vi "Aktualizacja ostatniego zaznaczonego położenia na mapie.vi"(6 "Pocz. poł.":T1 {"UTM"."N [m]" format="%#_10g"}, 7 "Aktualne położenie":T2 {"Szerokośc geograficzna - GPS" format="%_9f"; "Długość geograficzna - GPS" format="%_9f"; "Położenie \nrobota  UTM"."E [m]" format="%#_10g"; "Położenie \nrobota  UTM"."N [m]" format="%#_12g"}, 8 "Właściwości mapy in":T5, 9 "Mouse down coords":T3, 10 "Parametry odwzorowania Ziemi (WGS84)":cluster{"a":dbl, "b":dbl}, 11 "Picture in":refnum<vi>) -> (2 "Właściwości mapy out":T5, 3 "Pocz. poł. 2":T1 {"UTM"."N [m]" format="%#_10g"})   [LabVIEW 2012, in "Biblioteka moduł map v3.lvlib" / "Pomocnicze.lvlib"]
uses:
  Pomocnicze.lvlib
  <vilib>/Utility/miscctls.llb/LVBoundsTypeDef.ctl
  <vilib>/Utility/miscctls.llb/LVPoint32TypeDef.ctl
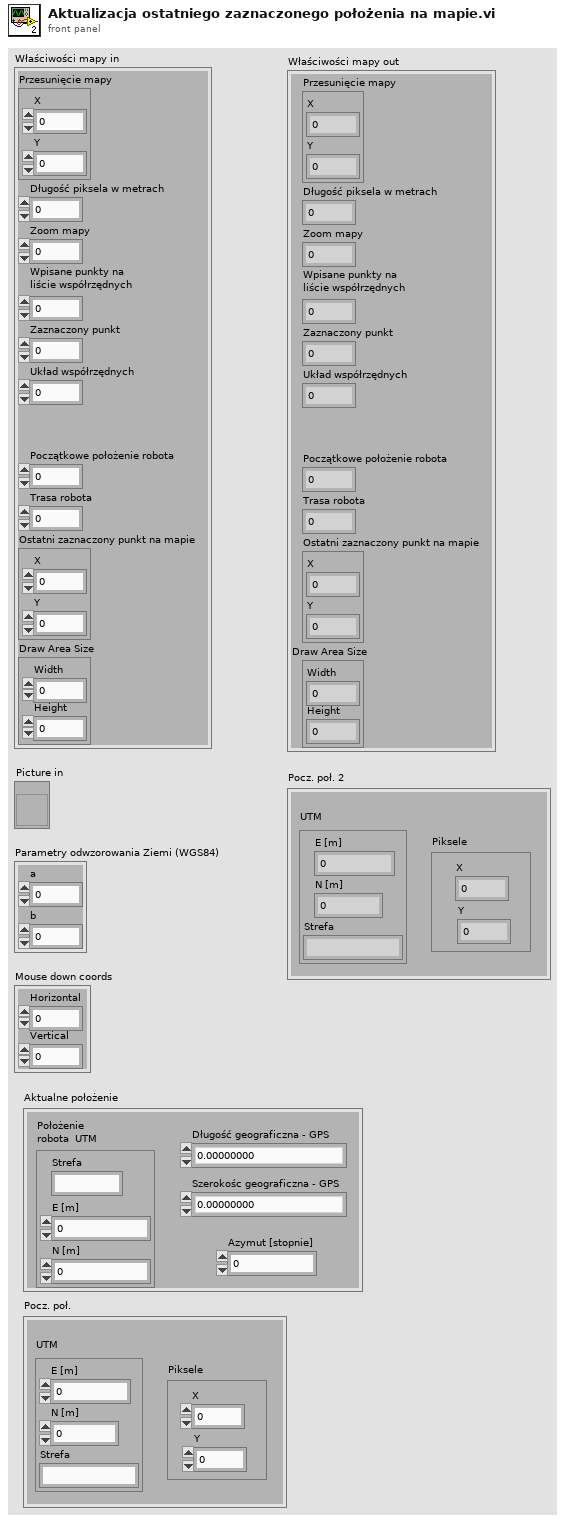
[diagram p1: front panel]
types:
  T1 = cluster{"UTM":cluster{"E [m]":ext, "N [m]":ext, "Strefa":string}, "Piksele":cluster{"X":i32, "Y":i32}}
  T2 = cluster{"Położenie \nrobota  UTM":cluster{"E [m]":ext, "N [m]":ext, "Strefa":string}, "Długość geograficzna - GPS":dbl, "Szerokośc geograficzna - GPS":dbl, "Azymut [stopnie]":dbl}
  T3 = typedef "LVPoint32TypeDef.ctl" = cluster{"Horizontal":i32, "Vertical":i32}
  T4 = typedef "LVBoundsTypeDef.ctl" = cluster{"Width":u32, "Height":u32}
  T5 = cluster{"Przesunięcie mapy":cluster{"X":i16, "Y":i16}, "Długość piksela w metrach":dbl, "Zoom mapy":sgl, "Wpisane punkty na\nliście współrzędnych":u32, "Zaznaczony punkt":u32, "Układ współrzędnych":u32, "Początkowe położenie robota":u32, "Trasa robota":u32, "Ostatni zaznaczony punkt na mapie":cluster{"X":i32, "Y":i32}, "Draw Area Size":T4}
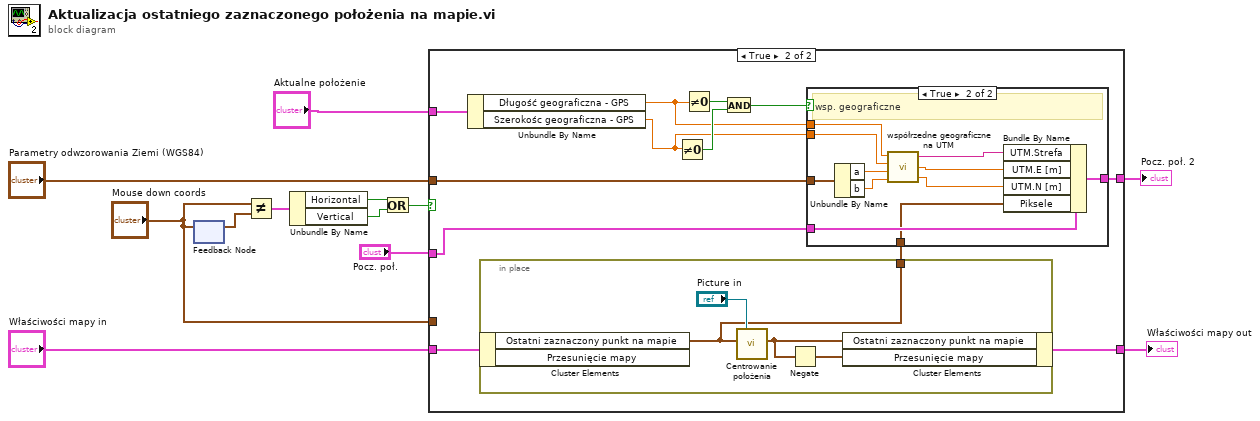
[diagram p0: block diagram]
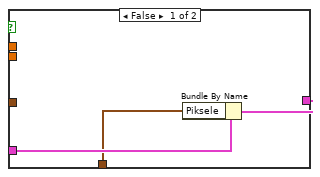
[diagram p3: hidden frame]
diagram:
  n1 = feedback #1() -> (w5:T3)  [unwired: 1 in]
  n2 = feedback-in #1("Mouse down coords") -> ()
  n3 = Not Equal?(x="Mouse down coords", y=w5) -> (x != y?=w6:cluster{"Horizontal":bool, "Vertical":bool})
  n4 = Unbundle By Name(w6) -> ("Horizontal"=w8:bool, "Vertical"=w9:bool)
  n5 = Or(x=w8, y=w9) -> (x .or. y?=w7:bool)
  n6 = case shown="True" w7 {
    tunnel: "Mouse down coords" -> [_ _]
    tunnel: "Właściwości mapy in" -> [w13 w17]
    tunnel: [w13 w19] -> w12
    tunnel: "Parametry odwzorowania Ziemi (WGS84)" -> [_ w26]
    tunnel: "Pocz. poł." -> [w14 w15]
    tunnel: [w14 w20] -> w1
    tunnel: "Aktualne położenie" -> [_ w16]
    frame False {
    }
    frame True {
      n7 = Unbundle By Name(w16) -> ("Długość geograficzna - GPS"=w21:dbl, "Szerokośc geograficzna - GPS"=w23:dbl)
      n8 = in-place {
        in-place-border: [w27] -> w18
        n9 = in-place-cluster #2(w17) -> ("Ostatni zaznaczony punkt na mapie"=w27:cluster{"X":i32, "Y":i32})  [unwired: 1 out]
        n10 = call "Centrowanie położenia.vi"("Ostatnie położenie robota"=w27, "Mapa z wprowadzonym punktem"="Picture in") -> ("Przesunięcie wycentrowane"=w28:T3)  [unwired: 9 in]
        n11 = Negate(x=w28) -> (-x=w29:T3)
        n12 = in-place-cluster #2("Ostatni zaznaczony punkt na mapie"=w28, "Przesunięcie mapy"=w29) -> (w19:T5)
      }
      n13 = Not Equal To 0?(x=w23) -> (x != 0?=w25:bool)
      n14 = Not Equal To 0?(x=w21) -> (x != 0?=w22:bool)
      n15 = And(x=w22, y=w25) -> (x .and. y?=w24:bool)
      n16 = case shown="True" w24 {
        tunnel: w26 -> [_ w44]
        tunnel: w21 -> [_ w38]
        tunnel: w23 -> [_ w37]
        tunnel: w15 -> [w33 w35]
        tunnel: [w31 w36] -> w20
        tunnel: w18 -> [w32 w34]
        frame False {
          n17 = Bundle By Name(cluster=w33, "Piksele"=w32) -> (w31:T1)
        }
        frame True {
          # "wsp. geograficzne"
          n18 = Unbundle By Name(w44) -> ("a"=w42:dbl, "b"=w43:dbl)
          n19 = call "współrzedne geograficzne na UTM.vi"("Położenie robota - długość geograficzna"=w38, "Położenie robota - szerokość geograficzna"=w37, "a"=w42, "b"=w43) -> ("Strefa"=w41:string, "E"=w40:ext, "N"=w39:ext)  [unwired: 2 in]
          n20 = Bundle By Name(cluster=w35, "UTM.Strefa"=w41, "UTM.E [m]"=w40, "UTM.N [m]"=w39, "Piksele"=w34) -> (w36:T1)
        }
      }
    }
  }
  "Właściwości mapy out" <- w12
  "Pocz. poł. 2" <- w1
